vi "Emballage_BDD_lecture_CODE_GESTION_join.vi"(8 "error in":errorcluster, 11 "ID_ARTICLE_GPAO":string) -> (0 "error out":errorcluster, 1 "données":string[](array[string]), 2 "Colonne":string[](array[string])=["ID_ARTICLE_GPAO", "NOVALVE_FILTRE", "INDICE_PRODUIT", "AFFICHE_CODEBARRE_CLIENT", "MELANGE_LOT_POSSIBLE", "FAMILLE_VALVE", "REMARQUE"], 3 "tableauHeaders":string[][](array[string]))   [LabVIEW 2020]
uses:
  Modules/FS/60_FS_Controles/60_FS_SetGet.ctl
  <vilib>/addons/database/Connection.llb/DB Tools Open Connec (Path).vi
  <vilib>/addons/database/Connection.llb/Conn Execute.vi
  <vilib>/addons/database/Recordset.llb/Rec Fetch Recordset Data (R).vi
  <vilib>/addons/database/Recordset.llb/Rec Destroy - Connection.vi
  <vilib>/addons/database/NI_Database_API.lvlib
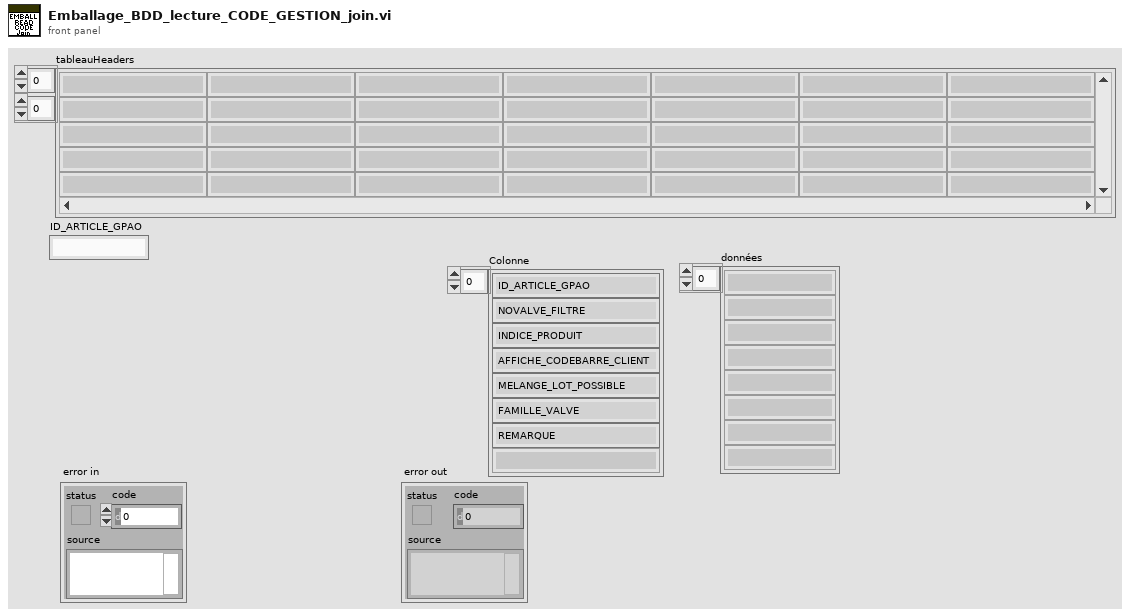
[diagram p1: front panel]
types:
  T1 = typedef "60_FS_SetGet.ctl" = enum16{"set", "get"}
  T2 = typedef "60_FS_CLT_Chemins.ctl" = cluster{"Racine_local":path, "Racine_reseau":path, "Racine_Support_Application":path, "Fichier_Journalisation":path, "Connexion_BDD_VSX":path, "Connexion_BDD_PLZ":path}
  T3 = typedef "NI_Database_API.lvlib/Conn ObjectReference.ctl" = refnum<k1>
  T4 = typedef "NI_Database_API.lvlib/Rec ObjectReference.ctl" = refnum<k1>
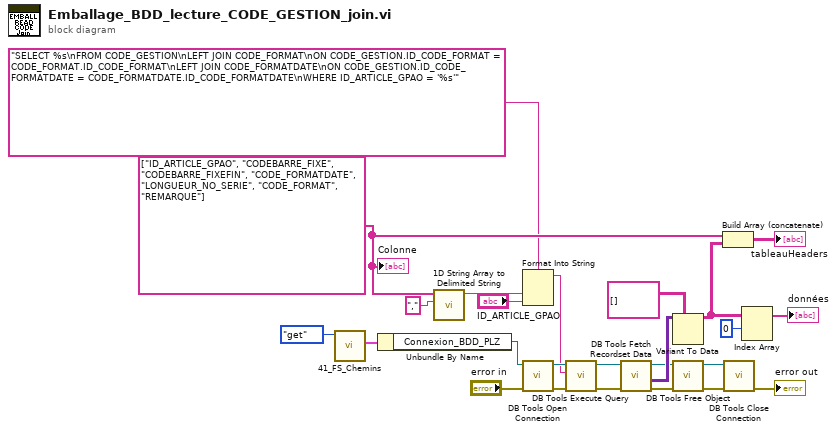
[diagram p0: block diagram]
diagram:
  w9 = string[] ["ID_ARTICLE_GPAO", "CODEBARRE_FIXE", "CODEBARRE_FIXEFIN", "CODE_FORMATDATE", "LONGUEUR_NO_SERIE", "CODE_FORMAT", "REMARQUE"]
  n1 = call "41_FS_Chemins.vi"("SetGet"=60_FS_SetGet."get") -> ("CLT_Chemins_out"=w11:T2)  [unwired: 9 in, 1 out]
  n2 = Unbundle By Name(w11) -> ("Connexion_BDD_PLZ"=w10:path)
  n3 = call <vilib>:"1D String Array to Delimited String.vi"("delimiter"=",", "string array"=w9) -> ("delimited string"=w5:string)  [unwired: 9 in]
  n4 = Format Into String(format string="SELECT %s\nFROM CODE_GESTION\nLEFT JOIN CODE_FORMAT\nON CODE_GESTION.ID_CODE_FORMAT = CODE_FORMAT.ID_CODE_FORMAT\nLEFT JOIN CODE_FORMATDATE\nON CODE_GESTION.ID_CODE_FORMATDATE = CODE_FORMATDATE.ID_CODE_FORMATDATE\nWHERE ID_ARTICLE_GPAO = '%s'" ("SQL query"), w5, "ID_ARTICLE_GPAO") -> (resulting string=w7:string)  [unwired: 2 in, 1 out]
  n5 = call-poly <vilib>:"DB Tools Open Connection.vi"("error in (no error)"="error in", "connection information"=w10) -> ("error out"=w14:errorcluster, "connection reference"=w15:T3)  [unwired: 6 in]
  n6 = call-poly <vilib>:"DB Tools Execute Query.vi"("error in (no error)"=w14, "SQL query"=w7, "connection reference"=w15) -> ("error out"=w24:errorcluster, "recordset reference"=w16:T4)  [unwired: 5 in]
  n7 = call-poly <vilib>:"DB Tools Fetch Recordset Data.vi"("error in (no error)"=w24, "recordset reference"=w16) -> ("error out"=w19:errorcluster, "recordset data"=w23:variant[][], "recordset reference out"=w20:T4)  [unwired: 3 in]
  n8 = Variant To Data(type=string[][] [] ("Liste des champs à lire 2"), Variant=w23) -> (data=w1:string[][])  [unwired: 1 in, 1 out]
  n9 = call-poly <vilib>:"DB Tools Free Object.vi"("error in (no error)"=w19, "recordset reference"=w20) -> ("error out"=w18:errorcluster, "connection reference"=w17:T3)  [unwired: 8 in]
  n10 = Build Array (concatenate)(w9, w1) -> (→"tableauHeaders":string[][])
  n11 = call <vilib>:"DB Tools Close Connection.vi"("error in (no error)"=w18, "connection reference"=w17) -> ("error out"=→"error out":errorcluster)  [unwired: 5 in]
  n12 = Index Array(array=w1, index (row)=0 ("indice (ligne)")) -> (element=→"données":string[])  [unwired: 1 in]
  "Colonne" <- w9
